vi "multiplicationTable.vi"() -> ()   [LabVIEW 2021]
panel:
  out "transposed array":dbl[][](array[numeric])
  in  "Start":dbl
  in  "End":dbl
  out "Array 2":dbl[][](array[numeric])
  out "Array":dbl[](array[numeric])
  in  "Numeric":dbl
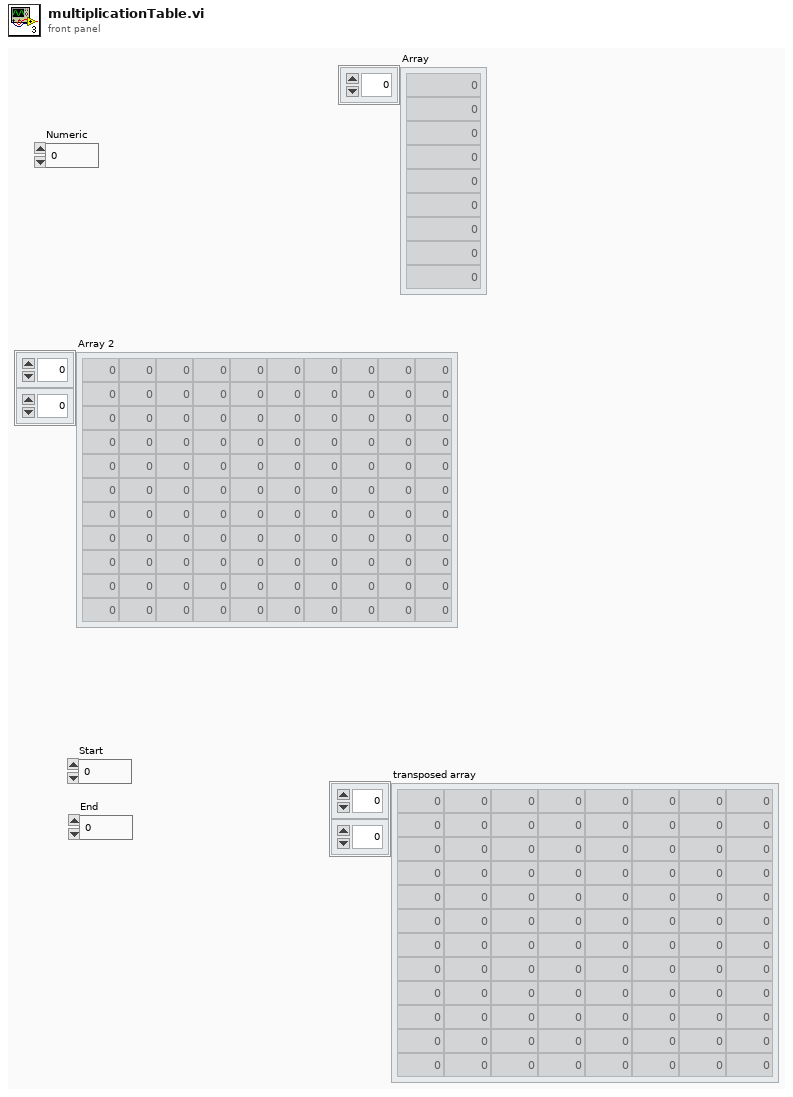
[diagram p1: front panel]
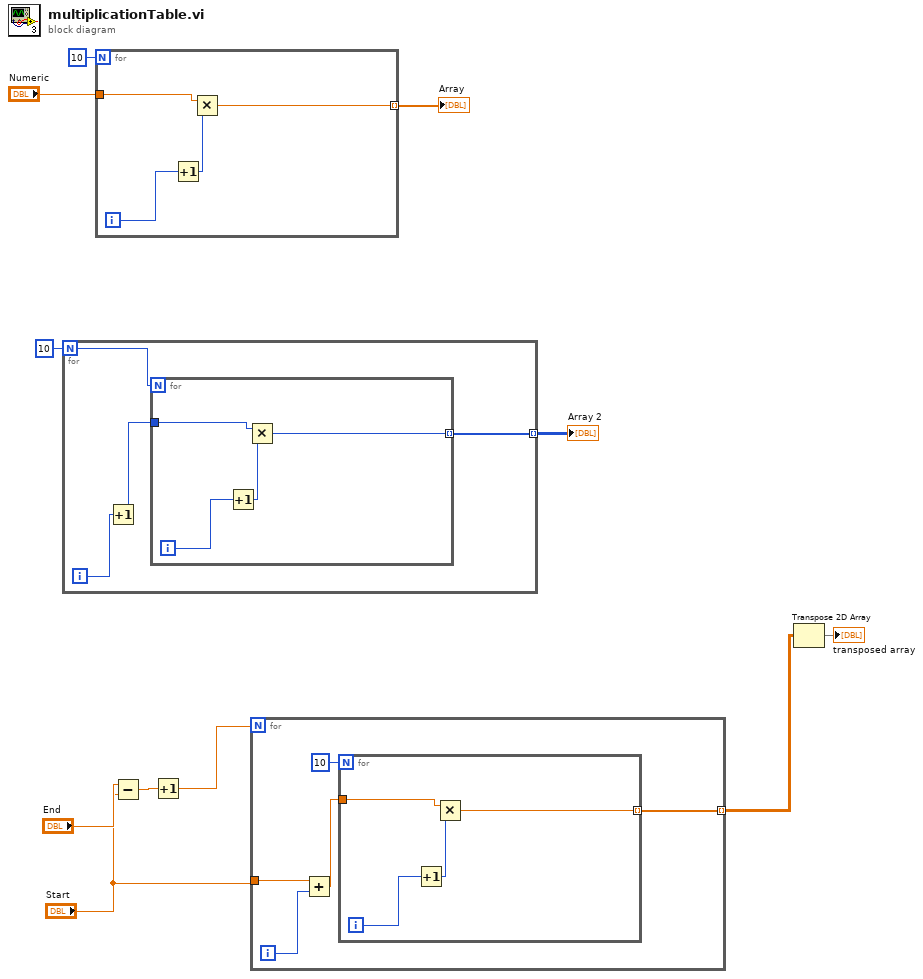
[diagram p0: block diagram]
diagram:
  n1 = for {
    N: 10 -> [w14]
    tunnel: [w15] -> w8 mode=indexing
    i -> [w13]
    n2 = Increment(x=w13) -> (x+1=w12:i32)
    n3 = for {
      N: w14 -> [_]
      tunnel: w12 -> [w19]
      tunnel: [w16] -> w15 mode=indexing
      i -> [w18]
      n4 = Increment(x=w18) -> (x+1=w17:i32)
      n5 = Multiply(x=w19, y=w17) -> (x*y=w16:i32)
    }
  }
  "Array 2" <- w8
  n6 = for {
    N: 10 -> [_]
    tunnel: "Numeric" -> [w23]
    tunnel: [w20] -> w9 mode=indexing
    i -> [w22]
    n7 = Increment(x=w22) -> (x+1=w21:i32)
    n8 = Multiply(x=w23, y=w21) -> (x*y=w20:dbl)
  }
  "Array" <- w9
  n9 = Subtract(x="End", y="Start") -> (x-y=w6:dbl)
  n10 = Increment(x=w6) -> (x+1=w5:dbl)
  n11 = for {
    N: w5 -> [_]
    tunnel: [w28] -> w3 mode=indexing
    tunnel: "Start" -> [w25]
    i -> [w26]
    n12 = Add(x=w25, y=w26) -> (x+y=w24:dbl)
    n13 = for {
      N: 10 -> [_]
      tunnel: w24 -> [w32]
      tunnel: [w29] -> w28 mode=indexing
      i -> [w31]
      n14 = Increment(x=w31) -> (x+1=w30:i32)
      n15 = Multiply(x=w32, y=w30) -> (x*y=w29:dbl)
    }
  }
  n16 = Transpose 2D Array(2D array=w3) -> (transposed array=→"transposed array":dbl[][])
